vi "Patrick Builder.vi"() -> ()   [LabVIEW 2019, in "Build.lvlib"]
uses:
  Build.lvlib
  <vilib>/Utility/sysdir.llb/System Directory Type.ctl
  Typedefs/Build Type--enum.ctl
  <vilib>/Hampel Software Engineering/Git API/Git API/GIT-api.lvclass
  <vilib>/Utility/file.llb/Read Delimited Spreadsheet (string).vi
  <vilib>/Utility/file.llb/Write Delimited Spreadsheet (string).vi
  <vilib>/regexp/Match Regular Expression.xnode
  <vilib>/JKI/VIPM API/VIPM API_vipm_api.lvlib
  VIPM/VIPM.lvlib
  Git/Git.lvclass
  <userlib>/_OpenG.lib/array/array.llb/Index 1D Array Elements (Path)__ogtk.vi
panel:
  in  "Open Repo":bool
  out "Mode":string
  in  "Edit build.cfg":bool
  in  "Edit Inno.iss":bool
  in  "Init Inno":bool
  in  "BAT File":path
  in  "Execute .bat":bool
  out "Output":string
  in  "Minor +1":bool
  in  "BAT":bool
  out "tag prefix":string caption="tag prefix (level1/level2)"
  in  "Edit File List":bool
  in  "Clear Notes":bool
  in  "Release Notes":string
  in  "Append Notes":bool
  in  "Patch +1":bool
  out "Selected File List":string
  out "Publish":bool
  in  "Open List":bool
  out "Build":bool
  in  "Preview":bool
  out "Status":string
  in  "File List":i32[](listbox)
  out "Package Builder":string
  # "Repository Config"
  # "Global Options (Applied to all Files)"
  # "Release Version"
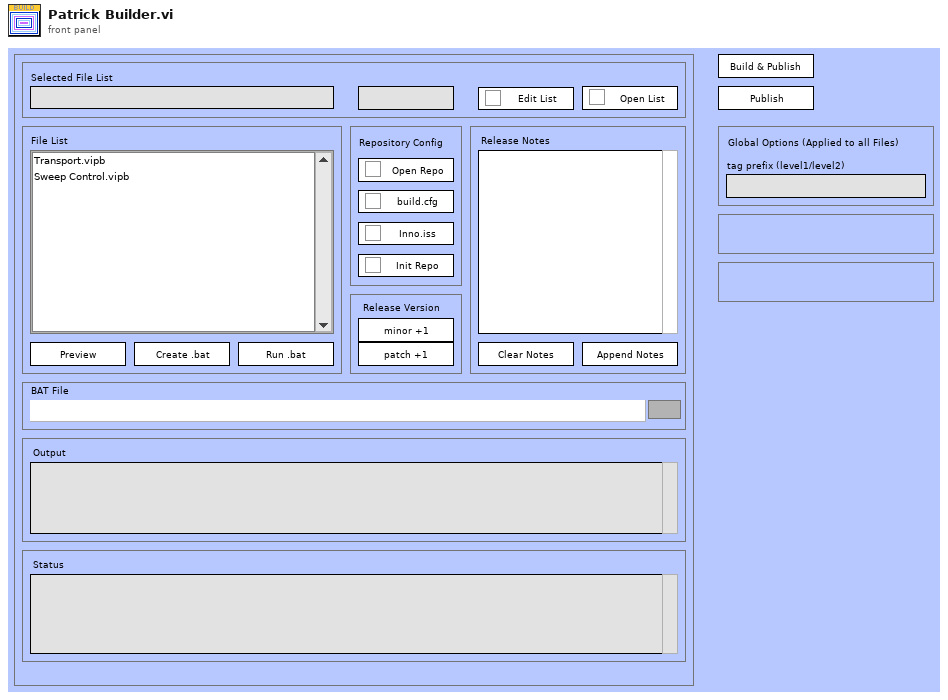
[diagram p1: front panel]
types:
  T1 = enum32{"Invalid", "Standard", "Closed", "Hidden", "Minimized", "Maximized"}
  T2 = enum32{"invalid app kind", "Development System", "Run Time System", "Student Edition", "Embedded LabVIEW", "Evaluation", "Custom"}
  T3 = enum8{"Enabled", "Disabled", "Disabled and Grayed Out"}
  T4 = typedef "Build.lvlib/Build Type--enum.ctl" = enum16{"Project (lvproj)", "Build Spec (vipb)", "Package (vip)"}
  T5 = cluster{"Core":cluster{"Current VI Reference":refnum<vi>, "Close Panel on Exit?":bool}, "lvproj paths":path[], "vipb paths":path[], "vip paths":path[], "selected paths":path[], "repository paths":path[], "path to open":path, ".bat path":path, "config folder":path, "config path":path, "Mode":T4, "git-api":refnum<class "GIT-api.lvclass">}
  T6 = typedef "System Directory Type.ctl" = i32
  T7 = cluster{"Current VI Reference":refnum<vi>, "Close Panel on Exit?":bool}
  T8 = typedef "VIPM API_vipm_api.lvlib/VI Package Build Spec Data Cluster_vipm_api.ctl" = cluster{"Package Version":T9, "Product Name":string, "Company Name":string, "Author Name (Person or Company)":string, "Product Homepage (URL)":string, "Legal Copyright":string, "License Agreement Name":string, "Product Description Summary":string, "Product Description":string, "Release Notes - Change Log":string}
  T9 = typedef "VIPM API_vipm_api.lvlib/Version Info Cluster_vipm_api.ctl" = cluster{"major":u32, "minor":u32, "patch":u32, "build":u32}
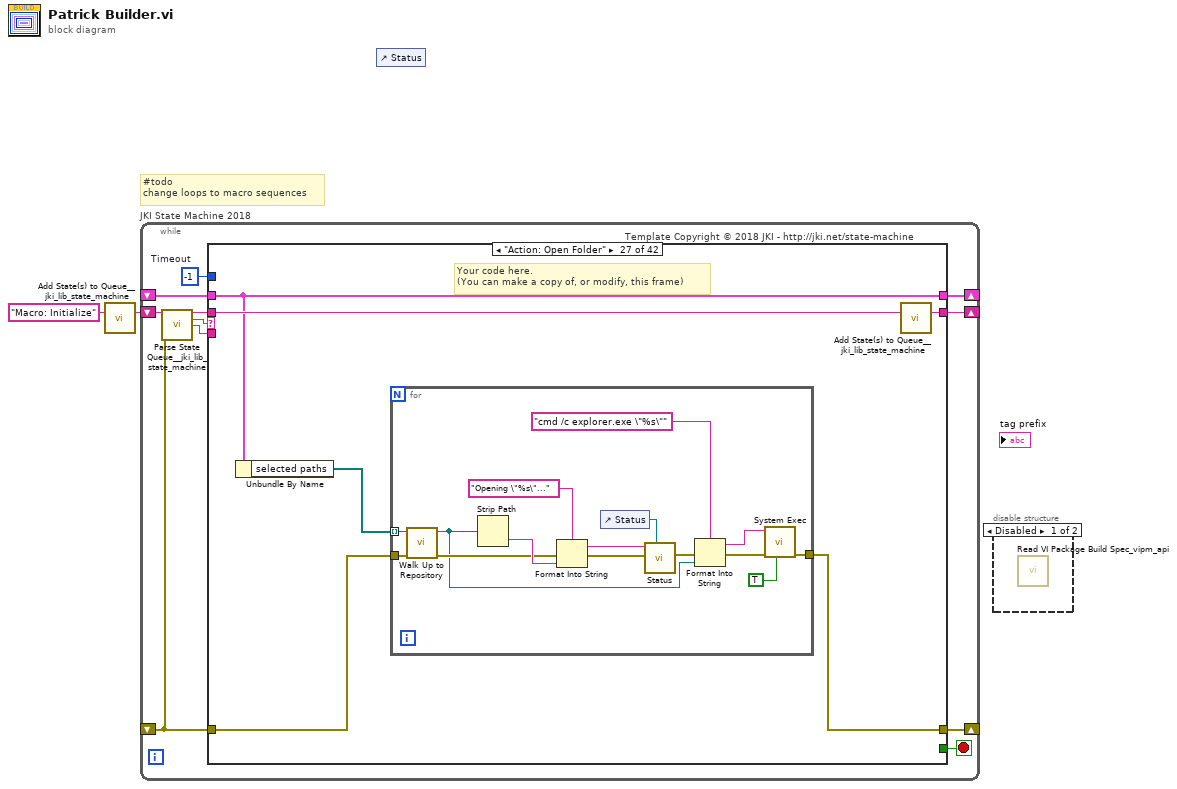
[diagram p0: block diagram]
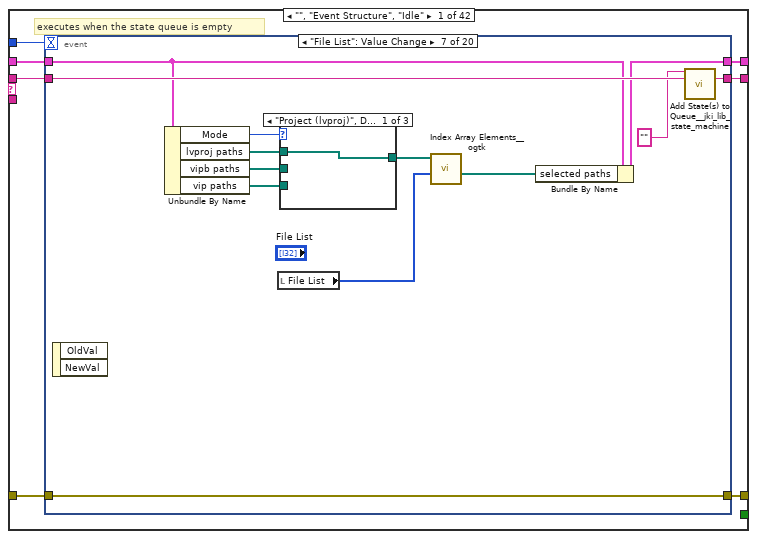
[diagram p3: hidden frame]
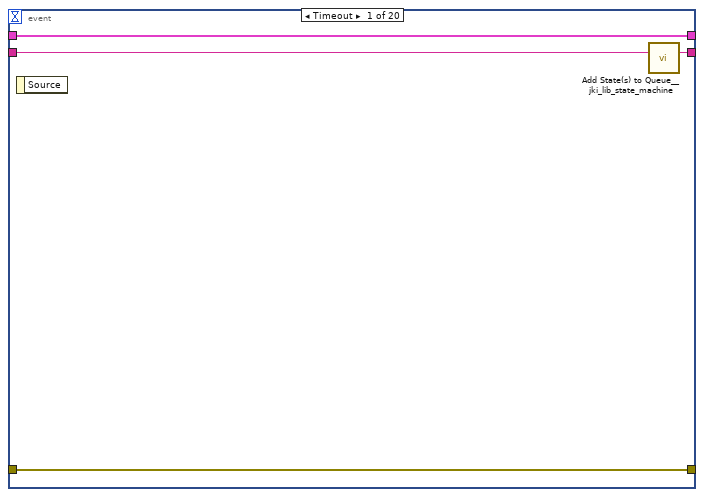
[diagram p4: hidden frame]
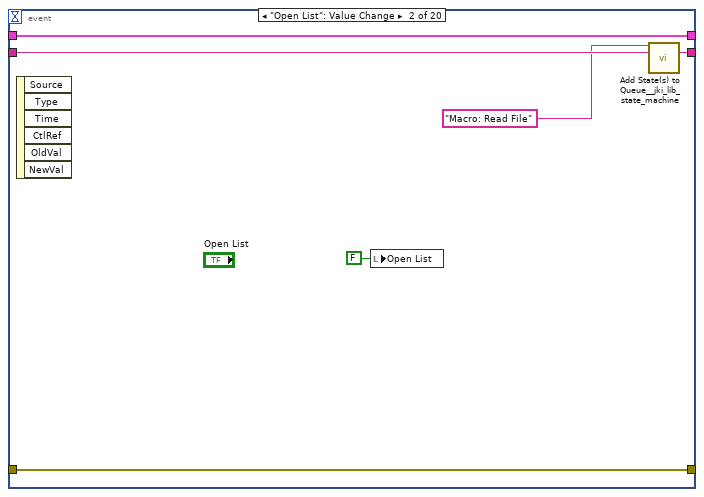
[diagram p5: hidden frame]
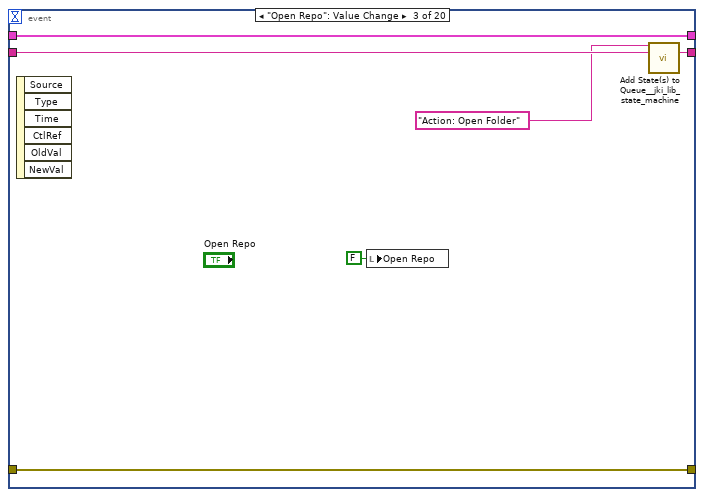
[diagram p6: hidden frame]
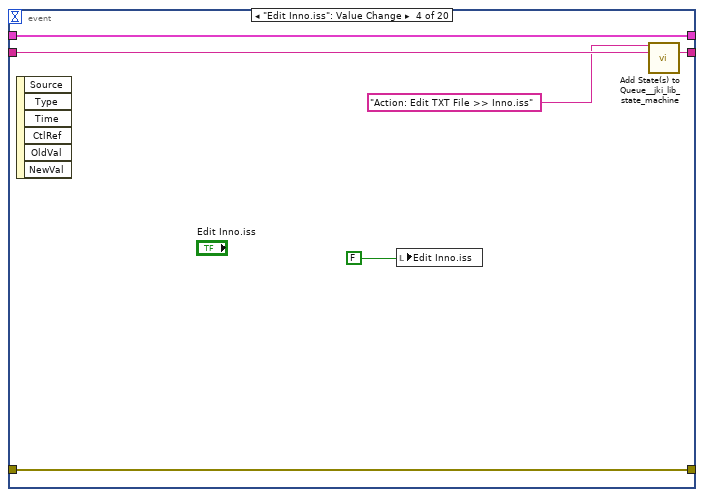
[diagram p7: hidden frame]
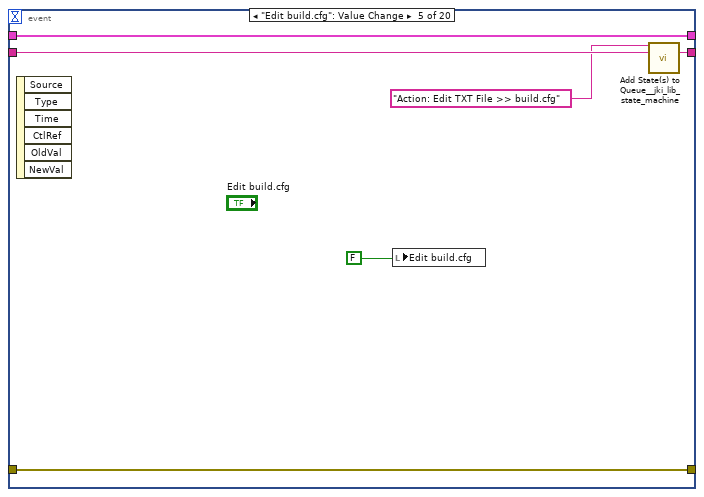
[diagram p8: hidden frame]
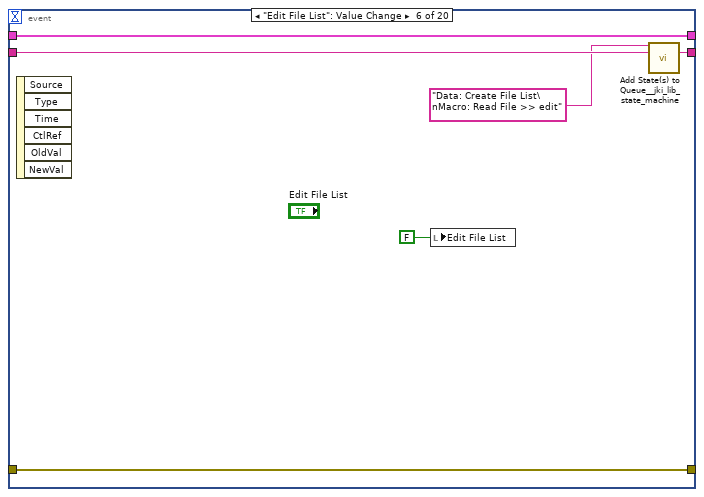
[diagram p9: hidden frame]
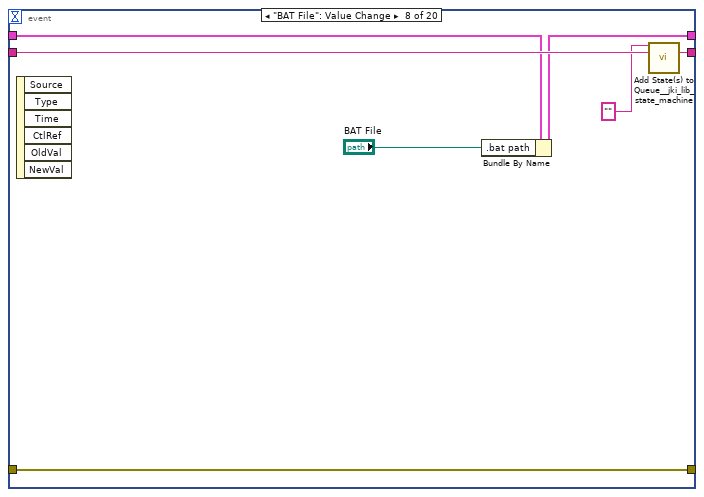
[diagram p12: hidden frame]
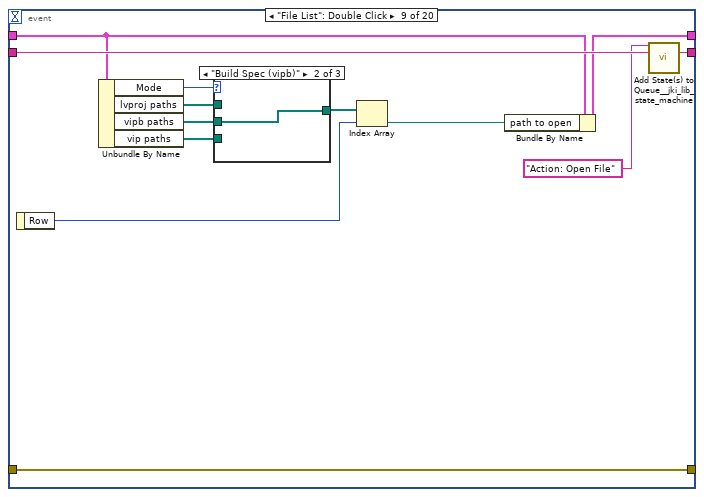
[diagram p13: hidden frame]
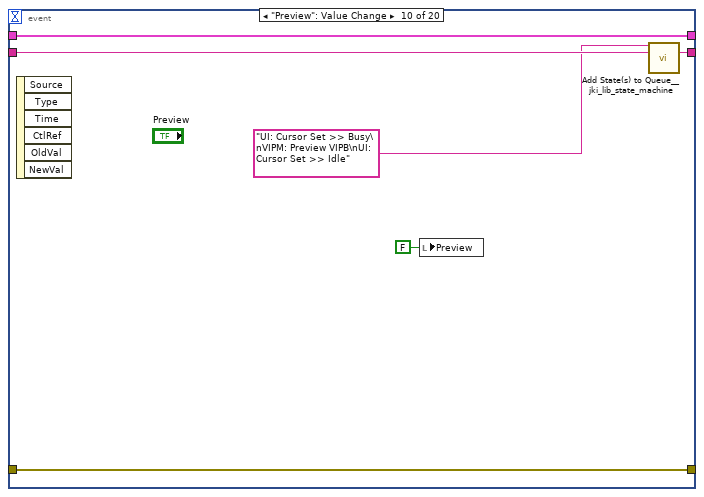
[diagram p16: hidden frame]
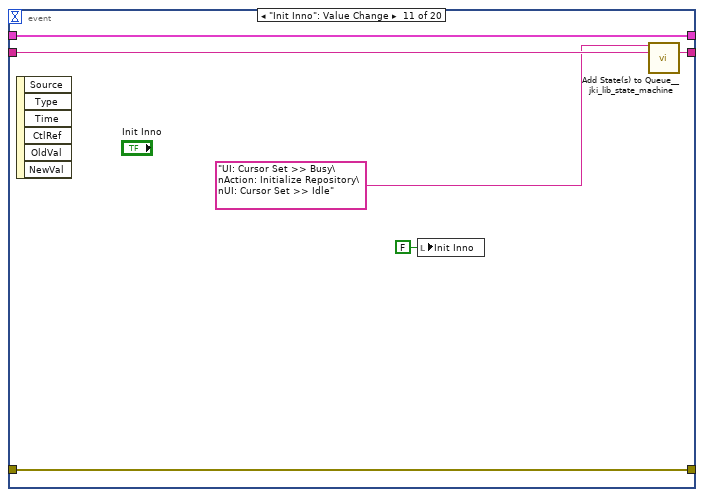
[diagram p17: hidden frame]
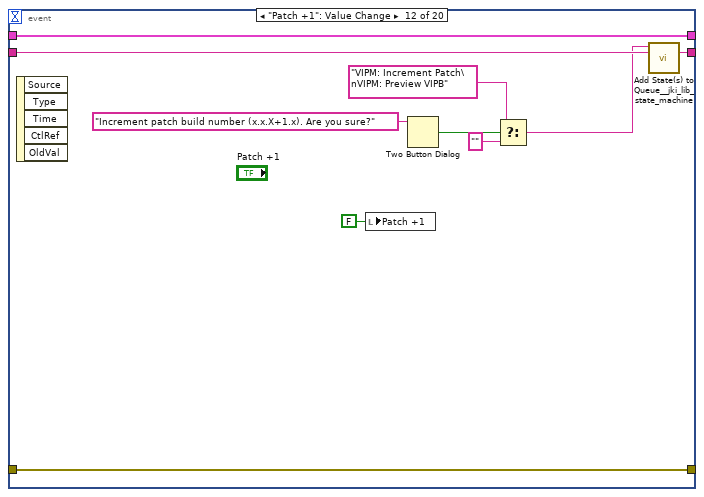
[diagram p18: hidden frame]
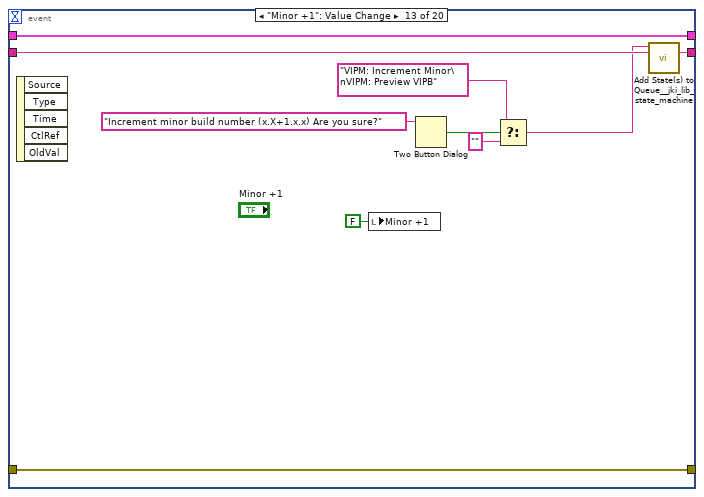
[diagram p19: hidden frame]
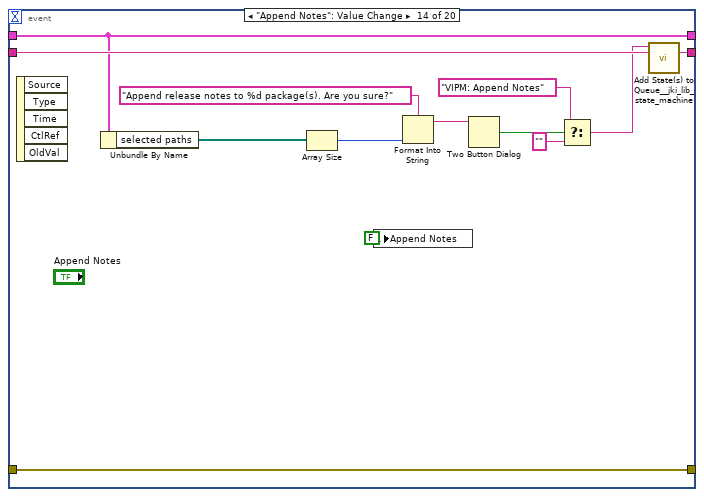
[diagram p20: hidden frame]
diagram:
  # "#todo\nchange loops to macro sequences"
  n1 = call <vilib>:"Add State(s) to Queue__jki_lib_state_machine.vi"("State(s) in (\"\")"="Macro: Initialize") -> ("States Out"=w2:string)  [unwired: 14 in]
  n2 = while "JKI State Machine 2018" {
    shift-right: [w7] -> _
    shift-left: _ -> [w6]
    shift-right: [w10] -> _
    shift-left: _ -> [w4]
    shift-right: [w9] -> _
    shift-left: w2 -> [w11]
    stop <- w8 stop-if-true
    w5 = -1  # Timeout
    # "Template Copyright © 2018 JKI - http://jki.net/state-machine"
    n3 = call <vilib>:"Parse State Queue__jki_lib_state_machine.vi"("State Queue"=w11, "Error In (no error)"=w4) -> ("Remaining States"=w13:string, "Current State"=w3:string, "Arguments"=w12:string)  [unwired: 11 in]
    n4 = case shown="\"Action: Open Folder\"" w3 {
      selector: w3 -> [_ _ w193 _ _ _ _ _ _ _ _ _ _ _ _ _ _ _ _ _ _ _ _ _ _ _ _ _ _ _ _ _ _ _ _ _ _ _ _ _ _ _]
      tunnel: w13 -> [w20 w192 w197 w216 w223 w232 w236 w260 w266 w276 w298 w316 w348 w382 w386 w400 w415 w437 w450 w461 w530 w535 w545 w555 w559 w575 w581 w609 w627 w646 w655 w672 w686 w703 w724 w746 w778 w800 w822 w954 w976 w980]
      tunnel: w12 -> [_ _ _ _ _ _ _ _ _ _ _ _ _ _ _ _ _ _ w445 w455 _ _ w536 _ _ _ _ _ w622 _ _ _ _ _ _ _ _ _ _ _ _ _]
      tunnel: w6 -> [w18 w189 w195 w209 w220 w230 w233 _ w261 w270 w294 w310 w337 w380 w383 w390 w412 w432 w448 w457 w527 w532 w542 w552 w556 w573 w579 w607 w625 w643 w653 w670 w684 w701 w722 w743 w769 w790 w812 w952 w973 w977]
      tunnel: [w17 w190 w199 w213 errorcluster {"status"=FALSE, "code"=0, "source"=""} ("error out") w229 w234 w253 w262 w274 w293 w313 w338 w376 w384 w398 w413 w435 w446 w458 w528 w533 w543 w553 w557 w572 w577 w603 w623 w644 w648 w668 w682 w695 w715 w737 w772 w788 w801 w950 w974 w978] -> w10
      tunnel: w4 -> [w16 w190 w198 w213 w218 w229 w234 w252 w263 w274 w291 w314 w345 w377 w384 w397 w413 w435 w447 w459 w528 w533 w543 w553 w557 w571 w578 w606 w624 w644 w652 w669 w683 w700 w721 w738 w773 w795 w820 w948 w974 w978]
      tunnel: [w19 w191 w196 w215 w222 w231 w235 w259 w265 w275 w297 w315 w347 w381 w385 w399 w414 w436 w449 w460 w529 w534 w544 w554 w558 w574 w580 w608 w626 w645 w654 w671 w685 w702 w723 w745 w777 w799 w821 w953 w975 w979] -> w9
      tunnel: [_ _ _ _ _ TRUE _ _ _ _ _ _ _ _ _ _ _ _ _ _ _ _ _ _ _ _ _ _ _ _ _ _ _ _ _ _ _ _ _ _ _ _] -> w8
      tunnel: [w15 w189 w195 w214 w220 w230 w233 w258 w261 w272 w295 w312 w336 w380 w383 w390 w412 w432 w448 w457 w527 w532 w542 w552 w556 w573 w579 w607 w625 w643 w653 w670 w684 w701 w722 w744 w770 w791 w813 w952 w973 w977] -> w7
      tunnel: w5 -> [w14 _ _ _ _ _ _ _ _ _ _ _ _ _ _ _ _ _ _ _ _ _ _ _ _ _ _ _ _ _ _ _ _ _ _ _ _ _ _ _ _ _]
      frame "", "Event Structure", "Idle" {
        # "executes when the state queue is empty"
        n5 = event shown="[6] \"File List\": Value Change" {
          selector: _ -> [_ _ _ _ _ _ _ _ _ _ _ _ _ _ _ _ _ _ _ _]
          dyn-events: _ -> [_ _ _ _ _ _ _ _ _ _ _ _ _ _ _ _ _ _ _ _]
          timeout: w14 -> [_ _ _ _ _ _ _ _ _ _ _ _ _ _ _ _ _ _ _ _]
          tunnel: w20 -> [w24 w30 w36 w42 w48 w54 w67 w77 w90 w99 w105 w115 w125 w138 w151 w164 w170 w176 w182 w188]
          tunnel: [w23 w29 w35 w41 w47 w53 w66 w76 w89 w98 w104 w114 w124 w137 w150 w163 w169 w175 w181 w187] -> w19
          tunnel: w18 -> [w21 w26 w32 w38 w44 w50 w64 w74 w79 w96 w102 w112 w122 w130 w143 w157 w167 w173 w179 w185]
          tunnel: [w22 w27 w33 w39 w45 w51 w65 w75 w88 w97 w103 w113 w123 w136 w149 w162 w168 w174 w180 w186] -> w17
          tunnel: w16 -> [w22 w27 w33 w39 w45 w51 w65 w75 w88 w97 w103 w113 w123 w136 w149 w162 w168 w174 w180 w186]
          tunnel: [w21 w26 w32 w38 w44 w50 w63 w73 w87 w96 w102 w112 w122 w130 w143 w157 w167 w173 w179 w185] -> w15
          event Timeout {
            n6 = event-data() -> ()  [unwired: 1 in, 1 out]
            n7 = call <vilib>:"Add State(s) to Queue__jki_lib_state_machine.vi"("State(s) in (\"\")"=w24) -> ("States Out"=w23:string)  [unwired: 14 in]
          }
          event "Open List": Value Change {
            n8 = event-data() -> ()  [unwired: 1 in, 6 out]
            n9 = local write "Open List"(FALSE ("Open List")) -> ()
            n10 = call <vilib>:"Add State(s) to Queue__jki_lib_state_machine.vi"("State(s) in Front (\"\")"="Macro: Read File" ("State(s) in Front (\"\")"), "State(s) in (\"\")"=w30) -> ("States Out"=w29:string)  [unwired: 13 in]
          }
          event "Open Repo": Value Change {
            n11 = event-data() -> ()  [unwired: 1 in, 6 out]
            n12 = local write "Open Repo"(FALSE ("Open List")) -> ()
            n13 = call <vilib>:"Add State(s) to Queue__jki_lib_state_machine.vi"("State(s) in Front (\"\")"="Action: Open Folder" ("State(s) in Front (\"\")"), "State(s) in (\"\")"=w36) -> ("States Out"=w35:string)  [unwired: 13 in]
          }
          event "Edit Inno.iss": Value Change {
            n14 = event-data() -> ()  [unwired: 1 in, 6 out]
            n15 = local write "Edit Inno.iss"(FALSE ("Open List")) -> ()
            n16 = call <vilib>:"Add State(s) to Queue__jki_lib_state_machine.vi"("State(s) in Front (\"\")"="Action: Edit TXT File >> Inno.iss" ("State(s) in Front (\"\")"), "State(s) in (\"\")"=w42) -> ("States Out"=w41:string)  [unwired: 13 in]
          }
          event "Edit build.cfg": Value Change {
            n17 = event-data() -> ()  [unwired: 1 in, 6 out]
            n18 = local write "Edit build.cfg"(FALSE ("Open List")) -> ()
            n19 = call <vilib>:"Add State(s) to Queue__jki_lib_state_machine.vi"("State(s) in Front (\"\")"="Action: Edit TXT File >> build.cfg" ("State(s) in Front (\"\")"), "State(s) in (\"\")"=w48) -> ("States Out"=w47:string)  [unwired: 13 in]
          }
          event "Edit File List": Value Change {
            n20 = event-data() -> ()  [unwired: 1 in, 6 out]
            n21 = local write "Edit File List"(FALSE ("Create File List")) -> ()
            n22 = call <vilib>:"Add State(s) to Queue__jki_lib_state_machine.vi"("State(s) in Front (\"\")"="Data: Create File List\nMacro: Read File >> edit" ("State(s) in Front (\"\")"), "State(s) in (\"\")"=w54) -> ("States Out"=w53:string)  [unwired: 13 in]
          }
          event "File List": Value Change {
            n23 = event-data() -> ()  [unwired: 1 in, 2 out]
            n24 = Unbundle By Name(w64) -> ("Mode"=w60:T4, "lvproj paths"=w58:path[], "vipb paths"=w57:path[], "vip paths"=w59:path[])
            n25 = local read "File List"() -> (w56:i32[])
            n26 = case shown="\"Project (lvproj)\", Default" w60 {
              tunnel: [w68 w69 w70] -> w55
              tunnel: w59 -> [_ _ w70]
              tunnel: w58 -> [w68 _ _]
              tunnel: w57 -> [_ w69 _]
              frame "Project (lvproj)", Default {
              }
              frame "Build Spec (vipb)" {
              }
              frame "Package (vip)" {
              }
            }
            n27 = call-poly <userlib>:"Index Array Elements__ogtk.vi"("indices"=w56, "array"=w55) -> ("elements"=w62:path[])  [unwired: 9 in]
            n28 = Bundle By Name(cluster=w64, "selected paths"=w62) -> (w63:T5)
            n29 = call <vilib>:"Add State(s) to Queue__jki_lib_state_machine.vi"("State(s) in Front (\"\")"="" ("State(s) in Front (\"\")"), "State(s) in (\"\")"=w67) -> ("States Out"=w66:string)  [unwired: 13 in]
          }
          event "BAT File": Value Change {
            n30 = event-data() -> ()  [unwired: 1 in, 6 out]
            n31 = Bundle By Name(cluster=w74, ".bat path"="BAT File") -> (w73:T5)
            n32 = call <vilib>:"Add State(s) to Queue__jki_lib_state_machine.vi"("State(s) in Front (\"\")"="" ("State(s) in Front (\"\")"), "State(s) in (\"\")"=w77) -> ("States Out"=w76:string)  [unwired: 13 in]
          }
          event "File List": Double Click {
            n33 = event-data() -> ("Row"=w84:i32)  [unwired: 1 in]
            n34 = Unbundle By Name(w79) -> ("Mode"=w83:T4, "lvproj paths"=w81:path[], "vipb paths"=w80:path[], "vip paths"=w82:path[])
            n35 = case shown="\"Build Spec (vipb)\"" w83 {
              tunnel: [w91 w92 w93] -> w78
              tunnel: w82 -> [_ _ w93]
              tunnel: w81 -> [w91 _ _]
              tunnel: w80 -> [_ w92 _]
              frame "Project (lvproj)", Default {
              }
              frame "Build Spec (vipb)" {
              }
              frame "Package (vip)" {
              }
            }
            n36 = Index Array(array=w78, index=w84) -> (element=w86:path)
            n37 = Bundle By Name(cluster=w79, "path to open"=w86) -> (w87:T5)
            n38 = call <vilib>:"Add State(s) to Queue__jki_lib_state_machine.vi"("State(s) in Front (\"\")"="Action: Open File" ("State(s) in Front (\"\")"), "State(s) in (\"\")"=w90) -> ("States Out"=w89:string)  [unwired: 13 in]
          }
          event "Preview": Value Change {
            n39 = event-data() -> ()  [unwired: 1 in, 6 out]
            n40 = local write "Preview"(FALSE ("Preview")) -> ()
            n41 = call <vilib>:"Add State(s) to Queue__jki_lib_state_machine.vi"("State(s) in Front (\"\")"="UI: Cursor Set >> Busy\nVIPM: Preview VIPB\nUI: Cursor Set >> Idle" ("State(s) in Front (\"\")"), "State(s) in (\"\")"=w99) -> ("States Out"=w98:string)  [unwired: 13 in]
          }
          event "Init Inno": Value Change {
            n42 = event-data() -> ()  [unwired: 1 in, 6 out]
            n43 = local write "Init Inno"(FALSE ("Preview")) -> ()
            n44 = call <vilib>:"Add State(s) to Queue__jki_lib_state_machine.vi"("State(s) in Front (\"\")"="UI: Cursor Set >> Busy\nAction: Initialize Repository\nUI: Cursor Set >> Idle" ("State(s) in Front (\"\")"), "State(s) in (\"\")"=w105) -> ("States Out"=w104:string)  [unwired: 13 in]
          }
          event "Patch +1": Value Change {
            n45 = event-data() -> ()  [unwired: 1 in, 5 out]
            n46 = local write "Patch +1"(FALSE ("Patch +1")) -> ()
            n47 = Two Button Dialog(message="Increment patch build number (x.x.X+1.x). Are you sure?") -> (T button?=w110:bool)  [unwired: 2 in]
            n48 = Select(t="VIPM: Increment Patch\nVIPM: Preview VIPB" ("State(s) in Front (\"\")"), s=w110, f="") -> (s? t:f=w108:string)
            n49 = call <vilib>:"Add State(s) to Queue__jki_lib_state_machine.vi"("State(s) in Front (\"\")"=w108, "State(s) in (\"\")"=w115) -> ("States Out"=w114:string)  [unwired: 13 in]
          }
          event "Minor +1": Value Change {
            n50 = event-data() -> ()  [unwired: 1 in, 5 out]
            n51 = local write "Minor +1"(FALSE ("Patch +1")) -> ()
            n52 = Two Button Dialog(message="Increment minor build number (x.X+1.x.x) Are you sure?") -> (T button?=w120:bool)  [unwired: 2 in]
            n53 = Select(t="VIPM: Increment Minor\nVIPM: Preview VIPB" ("State(s) in Front (\"\")"), s=w120, f="") -> (s? t:f=w118:string)
            n54 = call <vilib>:"Add State(s) to Queue__jki_lib_state_machine.vi"("State(s) in Front (\"\")"=w118, "State(s) in (\"\")"=w125) -> ("States Out"=w124:string)  [unwired: 13 in]
          }
          event "Append Notes": Value Change {
            n55 = event-data() -> ()  [unwired: 1 in, 5 out]
            n56 = Unbundle By Name(w130) -> ("selected paths"=w128:path[])
            n57 = Array Size(array=w128) -> (size(s)=w129:i32)
            n58 = local write "Append Notes"(FALSE ("Patch +1")) -> ()
            n59 = Format Into String(format string="Append release notes to %d package(s). Are you sure?" ("message"), w129) -> (resulting string=w132:string)  [unwired: 2 in, 1 out]
            n60 = Two Button Dialog(message=w132) -> (T button?=w135:bool)  [unwired: 2 in]
            n61 = Select(t="VIPM: Append Notes" ("State(s) in Front (\"\")"), s=w135, f="") -> (s? t:f=w133:string)
            n62 = call <vilib>:"Add State(s) to Queue__jki_lib_state_machine.vi"("State(s) in Front (\"\")"=w133, "State(s) in (\"\")"=w138) -> ("States Out"=w137:string)  [unwired: 13 in]
          }
          event "Clear Notes": Value Change {
            n63 = event-data() -> ()  [unwired: 1 in, 6 out]
            n64 = Unbundle By Name(w143) -> ("selected paths"=w141:path[])
            n65 = local write "Clear Notes"(FALSE ("Patch +1")) -> ()
            n66 = Array Size(array=w141) -> (size(s)=w142:i32)
            n67 = Format Into String(format string="Clear release notes from %d package(s). Are you sure?" ("message"), w142) -> (resulting string=w145:string)  [unwired: 2 in, 1 out]
            n68 = Two Button Dialog(message=w145) -> (T button?=w148:bool)  [unwired: 2 in]
            n69 = Select(t="VIPM: Clear Notes" ("State(s) in Front (\"\")"), s=w148, f="") -> (s? t:f=w146:string)
            n70 = call <vilib>:"Add State(s) to Queue__jki_lib_state_machine.vi"("State(s) in Front (\"\")"=w146, "State(s) in (\"\")"=w151) -> ("States Out"=w150:string)  [unwired: 13 in]
          }
          event "Build": Value Change {
            n71 = event-data() -> ()  [unwired: 1 in, 6 out]
            n72 = Unbundle By Name(w157) -> ("selected paths"=w153:path[])
            n73 = local write "Build"(FALSE ("Patch +1")) -> ()
            n74 = Array Size(array=w153) -> (size(s)=w154:i32)
            n75 = Format Into String(format string="You have chosen to build and publish %d package(s). Are you sure?" ("message"), w154) -> (resulting string=w156:string)  [unwired: 2 in, 1 out]
            n76 = Two Button Dialog(message=w156) -> (T button?=w161:bool)  [unwired: 2 in]
            n77 = Select(t="VIPM: Build\nUI: Disable Buttons\nUI: Enable Buttons\nVIPM: Publish" ("State(s) in Front (\"\")"), s=w161, f="") -> (s? t:f=w158:string)
            n78 = call <vilib>:"Add State(s) to Queue__jki_lib_state_machine.vi"("State(s) in Front (\"\")"=w158, "State(s) in (\"\")"=w164) -> ("States Out"=w163:string)  [unwired: 13 in]
          }
          event "Publish": Value Change {
            n79 = event-data() -> ()  [unwired: 1 in, 6 out]
            n80 = local write "Publish"(FALSE ("Patch +1")) -> ()
            n81 = call <vilib>:"Add State(s) to Queue__jki_lib_state_machine.vi"("State(s) in Front (\"\")"="VIPM: Publish" ("State(s) in Front (\"\")"), "State(s) in (\"\")"=w170) -> ("States Out"=w169:string)  [unwired: 13 in]
          }
          event "BAT": Value Change {
            n82 = event-data() -> ()  [unwired: 1 in, 6 out]
            n83 = local write "BAT"(FALSE ("Patch +1")) -> ()
            n84 = call <vilib>:"Add State(s) to Queue__jki_lib_state_machine.vi"("State(s) in Front (\"\")"="VIPM: Create Build File\nVIPM: Create Build All File" ("State(s) in Front (\"\")"), "State(s) in (\"\")"=w176) -> ("States Out"=w175:string)  [unwired: 13 in]
          }
          event "Execute .bat": Value Change {
            n85 = event-data() -> ()  [unwired: 1 in, 6 out]
            n86 = local write "Execute .bat"(FALSE ("Patch +1")) -> ()
            n87 = call <vilib>:"Add State(s) to Queue__jki_lib_state_machine.vi"("State(s) in Front (\"\")"="VIPM: Run BAT File\nVIPM: Publish" ("State(s) in Front (\"\")"), "State(s) in (\"\")"=w182) -> ("States Out"=w181:string)  [unwired: 13 in]
          }
          event Panel Close? {
            # "Discard the event because we'll close the front panel ourselves in Macro: Exit"
            # "Close Panel button (pressed) Event\n(this executes Macro: Exit to terminate the VI)"
            n88 = event-data() -> ()  [unwired: 1 in, 1 out]
            n89 = event-data("Discard?"=TRUE) -> ()  [unwired: 1 in, 1 out]
            n90 = call <vilib>:"Add State(s) to Queue__jki_lib_state_machine.vi"("State(s) in Front (\"\")"="Macro: Exit", "State(s) in (\"\")"=w188) -> ("States Out"=w187:string)  [unwired: 13 in]
          }
        }
      }
      frame "---------- Core ----------" {
        # "Do not put any code in this frame.\n(it is a separator no-op)"
        n91 = call <vilib>:"Add State(s) to Queue__jki_lib_state_machine.vi"("State(s) in (\"\")"=w192) -> ("States Out"=w191:string)  [unwired: 14 in]
      }
      frame Default {
        w202 = 42 items=["No error", "Argument error", "Memory is full", "Out of zone", "End of file", "File already open", "Generic file I/O error", "File not found", "File permission error", "Disk is full", "Duplicate path", "Too many files open", "System feature not enabled", "Resource file not found", "Cannot add resource", "Resource not found", "Image not found", "Image memory error", "Pen does not exist", "Config type invalid", "Config token not found", "Config parse error", "Config memory error", "Bad external code format", "Bad external code offset", "External code not present", "Null window", "Destroy window error", "Null menu", "Print aborted", "Bad print record", "Print driver error", "Windows error during printing", "Memory error during printing", "Print dialog error", "Generic print error", "Invalid device refnum", "Device not found", "Device parameter error", "Device unit error", "Cannot open device", "Device call aborted", "Generic error", "Cancelled by user", "Object ID too low", "Object ID too high", "Object not in heap", "Unknown heap", "Unknown object (invalid DefProc)", "Unknown object (DefProc not in table)", "Message out of range", "Invalid (null) method", "Unknown message", "Manager call not supported", "Bad address", "Network operation in progress", "Network operation timed out", "Connection is busy", "Network attribute not supported", "Network error", "Address in use", "System out of memory", "Connection aborted", "Connection refused", "Not connected", "Already connected", "Connection closed", "Initialization error (interapplication manager)", "Bad occurrence", "Wait on unbound occurrence handler", "Occurrence queue overflow", "Datalog type conflict", "Unused", "Unrecognized type (interapplication manager)", "Memory corrupt", "Failed to make temporary DLL", "Old CIN version", "Drag socket not found", "Failed to load drop-object", "Failed to register OLE object", "Failed to release OLE object", "Format specifier type mismatch", "Unknown format specifier", "Too few format specifiers", "Too many format specifiers", "Scan failed", "Newer CIN version", "Error converting to variant", "Runtime menu error", "Password tampered", "Variant attribute not found", "Incompatible variant data type", "Event data is not available", "Event Store is not present", "Occurrence is not found", "Event Queue is not created", "Event info is not available", "Refnum passed is NULL", "Error retrieving Class GUID", "Error retrieving CoClass GUID", "Error retrieving TypeLib GUID.", "Bad built application magic bytes.", "Specific driver is different from the specific driver associated with the Logical Name.", "There is no session opened to the class driver.", "Max Error", "MAX - Error with config objects", "MAX - Error loading configuration", "MAX - Group not supported"]
        # "Current State"
        # "Do not delete, rename, or modify this frame.\n(this is used to capture unhandled states and typos)"
        # "Handle mistyped state name (developer tool)"
        n92 = Format Into String(format string="Software Exception: Unhandled State \"%s\"." ("message"), error in=w198, w193) -> (resulting string=w201:string, error out=w200:errorcluster)  [unwired: 1 in]
        n93 = call <vilib>:"Error Cluster From Error Code.vi"("show call chain? (False)"=TRUE, "error in (no error)"=w200, "error message (\"\")"=w201, "error code (0)"=w202) -> ("error out"=w199:errorcluster)  [unwired: 5 in]
        n94 = call <vilib>:"Add State(s) to Queue__jki_lib_state_machine.vi"("State(s) in (\"\")"=w197) -> ("States Out"=w196:string)  [unwired: 14 in]
      }
      frame "Initialize Core Data" {
        # "Do not delete, rename, or modify this frame.\n(this is used to determine panel behavior on exit)"
        # "originally closed?"
        # "exe?"
        # "If panel starts closed or is an EXE, then close it when we exit"
        n95 = property class="VI"() -> ("FP.State"=w206:T1)  [unwired: 2 in, 2 out]
        n96 = property class="App"() -> ("App.Kind"=w212:T2)  [unwired: 2 in, 2 out]
        n97 = control-ref of="Current VI Reference"() -> (w207:refnum<vi>)
        n98 = Equal?(x=w206, y=T1."Closed" ("Front Panel Window:State")) -> (x = y?=w204:bool)
        n99 = Equal?(x=w212, y=T2."Run Time System" ("Application:Kind")) -> (x = y?=w210:bool)
        n100 = Or(x=w204, y=w210) -> (x .or. y?=w208:bool)
        n101 = Bundle By Name(cluster=w209, "Core.Current VI Reference"=w207, "Core.Close Panel on Exit?"=w208) -> (w214:T5)
        n102 = call <vilib>:"Add State(s) to Queue__jki_lib_state_machine.vi"("State(s) in (\"\")"=w216) -> ("States Out"=w215:string)  [unwired: 14 in]
      }
      frame "Error Handler" {
        # "Unhandled Error -- Display it"
        # "Handle any errors here.\nYou can also output any states to clean-up after errors occur"
        # "Clear error"
        n103 = case shown="Default" w218 {
          selector: w218 -> [w224 w225 _]
          tunnel: [w224 w225 w226] -> w217
          frame No Error {
          }
          frame Default {
          }
          frame Error {
            n104 = property on="Open List" class="Bool (strict)"("Val(Sgnl)"=TRUE) -> (error out=w226:errorcluster)  [unwired: 2 in, 1 out]
          }
        }
        n105 = call <vilib>:"General Error Handler.vi"("error in (no error)"=w217) -> ()  [unwired: 10 in, 5 out]
        n106 = call <vilib>:"Add State(s) to Queue__jki_lib_state_machine.vi"("State(s) in Front (\"\")"="/* Post Error States", "State(s) in (\"\")"=w223) -> ("States Out"=w222:string)  [unwired: 13 in]
      }
      frame "Exit" {
        # "Do not put any code in this frame.\n(No errors that occur here will be handled.)"
        n107 = call <vilib>:"Add State(s) to Queue__jki_lib_state_machine.vi"("State(s) in (\"\")"=w232) -> ("States Out"=w231:string)  [unwired: 14 in]
      }
      frame "---------- Data ----------" {
        # "Do not put any code in this frame.\n(It is a separator no-op. You can make a copy of this frame to create a new Data frame)"
        n108 = call <vilib>:"Add State(s) to Queue__jki_lib_state_machine.vi"("State(s) in (\"\")"=w236) -> ("States Out"=w235:string)  [unwired: 14 in]
      }
      frame "Data: Initialize" {
        w237 = path ""  # .bat path
        w240 = path ""  # config folder
        w241 = path[] []  # repository paths
        w242 = path ""  # path to open
        w243 = refnum<class "GIT-api.lvclass"> refnum  # git-api
        w244 = Build_Type--enum."Project (lvproj)"  # Mode
        w248 = T6 3 items=["User Home"=0, "User Desktop"=1, "User Documents"=2, "User Application Data"=3, "User Preferences"=4, "User Temporary"=5, "Public Documents"=6, "Public Application Data"=7, "Public Preferences"=8, "Public Cache"=13, "System Core Libraries"=9, "System Installed Libraries"=10, "Application Files"=11, "Boot Volume Root"=12] ("system directory type")
        w249 = path[] []  # lvproj paths
        w250 = path[] []  # vip paths
        w251 = path[] []  # vipb paths
        w254 = path ""  # config path
        w256 = path[] []  # selected paths
        w257 = T7 {"Current VI Reference"=refnum, "Close Panel on Exit?"=FALSE}  # Core
        # "Initialize the shift-register data, here.\n(data names are defined by what you wire into the bundle function)"
        n109 = call <vilib>:"Get System Directory.vi"("system directory type"=w248) -> ("system directory"=w247:path)  [unwired: 10 in]
        n110 = Build Path(base path=w247, name or relative path="LevyLab\\build-support") -> (appended path=w246:path)
        n111 = call <vilib>:"Create Directory Recursive.vi"("error in (no error)"=w252, "directory"=w246) -> ("error out"=w253:errorcluster, "directory copy"=w239:path)  [unwired: 3 in, 1 out]
        n112 = Variant To Data(type=w240, Variant=w239) -> (data=w238:path)  [unwired: 1 in, 1 out]
        n113 = Variant To Data(type=w254, Variant=w239) -> (data=w255:path)  [unwired: 1 in, 1 out]
        n114 = Bundle("Core"=w257, "lvproj paths"=w249, "vipb paths"=w251, "vip paths"=w250, "selected paths"=w256, "repository paths"=w241, "path to open"=w242, ".bat path"=w237, "config folder"=w238, "config path"=w255, "Mode"=w244, "git-api"=w243) -> (w258:T5)  [unwired: 1 in]
        n115 = call <vilib>:"Add State(s) to Queue__jki_lib_state_machine.vi"("State(s) in (\"\")"=w260) -> ("States Out"=w259:string)  [unwired: 14 in]
      }
      frame "Data: Cleanup" {
        # "Cleanup any data and references, here.\n(this is called automatically, by the Macro: Exit)"
        n116 = Unbundle By Name(w261) -> ("Core.Current VI Reference"=w264:refnum<vi>)
        n117 = Close Reference(reference=w264, error in (no error)=w263) -> (error out=w262:errorcluster)
        n118 = call <vilib>:"Add State(s) to Queue__jki_lib_state_machine.vi"("State(s) in (\"\")"=w266) -> ("States Out"=w265:string)  [unwired: 14 in]
      }
      frame "Data: Update Listbox" {
        # "Do not put any code in this frame.\n(It is a separator no-op. You can make a copy of this frame to create a new Data frame)"
        n119 = Unbundle By Name(w270) -> ("Mode"=w271:T4)
        n120 = case shown="\"Package (vip)\"" w271 {
          tunnel: w270 -> [w278 w280 w282]
          tunnel: [w277 w279 w281] -> w269
          frame "Project (lvproj)", Default {
            n121 = Unbundle By Name(w278) -> ("lvproj paths"=w277:path[])
          }
          frame "Build Spec (vipb)" {
            n122 = Unbundle By Name(w280) -> ("vipb paths"=w279:path[])
          }
          frame "Package (vip)" {
            n123 = Unbundle By Name(w282) -> ("vip paths"=w281:path[])
          }
        }
        n124 = for {
          tunnel: w269 -> [w285] mode=indexing
          tunnel: [w284] -> w273 mode=indexing
          tunnel: [w283] -> _ mode=indexing
          i -> [w283]
          n125 = Strip Path(path=w285) -> (name=w284:string)  [unwired: 1 out]
        }
        n126 = Bundle By Name(cluster=w270, "selected paths"=path[] [] ("f")) -> (w272:T5)
        n127 = property on="File List" class="LstBox (strict)"("Item Names"=w273, "Value"=i32[] [] ("File List")) -> ()  [unwired: 2 in, 2 out]
        n128 = call <vilib>:"Add State(s) to Queue__jki_lib_state_machine.vi"("State(s) in (\"\")"=w276) -> ("States Out"=w275:string)  [unwired: 14 in]
      }
      frame "Data: Choose File List" {
        # "Do not put any code in this frame.\n(It is a separator no-op. You can make a copy of this frame to create a new Data frame)"
        n129 = Unbundle By Name(w294) -> ("config path"=w290:path)
        n130 = call "File Dialog2"("start path"=w290, "prompt"="Choose list file to open", "error in"=w291, "pattern (all files)"="*.txt") -> ("selected path"=w287:path, "cancelled"=w289:bool, "error out"=w288:errorcluster)  [unwired: 8 in, 1 out]
        n131 = case shown="False" w289 {
          tunnel: w287 -> [w299 _]
          tunnel: [w303 _] -> w296
          tunnel: [w302 w304] -> w295
          tunnel: w294 -> [w301 w304]
          tunnel: w288 -> [w300 _]
          tunnel: [w300 _] -> w293
          frame False {
            n132 = Bundle By Name(cluster=w301, "config path"=w299) -> (w302:T5)
            n133 = Strip Path(path=w299) -> (name=w303:string)  [unwired: 1 out]
          }
          frame True {
          }
        }
        "Selected File List" <- w296
        n134 = call <vilib>:"Add State(s) to Queue__jki_lib_state_machine.vi"("State(s) in (\"\")"=w298) -> ("States Out"=w297:string)  [unwired: 14 in]
      }
      frame "Data: Create File List" {
        # "Do not put any code in this frame.\n(It is a separator no-op. You can make a copy of this frame to create a new Data frame)"
        n135 = Unbundle By Name(w310) -> ("config path"=w309:path, "Mode"=w308:T4)
        n136 = call "File List Window.vi"("error in"=w314, "File Type"=w308, "Path"=w309) -> ("error out"=w313:errorcluster, "File Type out"=w307:T4, "files out"=w306:path[], "Path out"=w305:path)  [unwired: 5 in]
        n137 = Empty Array?(array=w306) -> (empty?=w311:bool)
        n138 = case shown="False" w311 {
          tunnel: [w319 w332] -> w312
          tunnel: w310 -> [w322 w332]
          tunnel: w307 -> [w317 _]
          tunnel: w306 -> [w321 _]
          tunnel: w305 -> [w318 _]
          frame False {
            n139 = case shown="\"Build Spec (vipb)\"" w317 {
              tunnel: [w325 w328 w331] -> w320
              tunnel: w322 -> [w324 w327 w330]
              tunnel: w321 -> [w323 w326 w329]
              frame "Project (lvproj)" {
                n140 = Bundle By Name(cluster=w324, "lvproj paths"=w323) -> (w325:T5)
              }
              frame "Build Spec (vipb)" {
                n141 = Bundle By Name(cluster=w327, "vipb paths"=w326) -> (w328:T5)
              }
              frame "Package (vip)" {
                n142 = Bundle By Name(cluster=w330, "vip paths"=w329) -> (w331:T5)
              }
            }
            n143 = Bundle By Name(cluster=w320, "Mode"=w317, "config path"=w318) -> (w319:T5)
          }
          frame True {
          }
        }
        n144 = call <vilib>:"Add State(s) to Queue__jki_lib_state_machine.vi"("State(s) in (\"\")"=w316) -> ("States Out"=w315:string)  [unwired: 14 in]
      }
      frame "Data: Read File List" {
        # "Do not put any code in this frame.\n(It is a separator no-op. You can make a copy of this frame to create a new Data frame)"
        n145 = Unbundle By Name(w337) -> ("config path"=w346:path)
        n146 = call-poly <vilib>:"Read Delimited Spreadsheet.vi"("file path (dialog if empty)"=w346, "error in (no error)"=w345, "transpose? (F)"=TRUE, "delimiter (\\t)"="\\n" ("delimiter (\\t)")) -> ("all rows"=w343:string[][], "error out"=w339:errorcluster)  [unwired: 6 in, 4 out]
        n147 = Index Array(array=w343) -> (element=w342:string[])  [unwired: 2 in]
        n148 = String To Path(string=w342) -> (path=w340:path[])
        n149 = for {
          tunnel: w340 -> [w372] mode=indexing
          tunnel: w339 -> [w371]
          tunnel: [w370] -> w338
          tunnel: [w368] -> w335 mode=indexing
          tunnel: [w367] -> w333
          n150 = call <vilib>:"Get File Extension.vi"("error in (no error)"=w371, "file"=w372) -> ("error out"=w370:errorcluster, "lowercase file extension"=w369:string, "dup file"=w368:path)  [unwired: 5 in, 2 out]
          n151 = call "Extension to Mode.vi"("lowercase file extension"=w369) -> ("Mode"=w367:T4)  [unwired: 10 in]
        }
        n152 = Empty Array?(array=w335) -> (empty?=w334:bool)
        n153 = case shown="False" w334 {
          tunnel: [w353 w366] -> w336
          tunnel: w337 -> [w352 w366]
          tunnel: w333 -> [w350 _]
          tunnel: w335 -> [w351 _]
          frame False {
            n154 = case shown="\"Package (vip)\"" w350 {
              selector: w350 -> [w354 w358 w362]
              tunnel: [w357 w361 w365] -> w353
              tunnel: w352 -> [w356 w360 w364]
              tunnel: w351 -> [w355 w359 w363]
              frame "Project (lvproj)" {
                n155 = Bundle By Name(cluster=w356, "lvproj paths"=w355, "Mode"=w354) -> (w357:T5)
              }
              frame "Build Spec (vipb)" {
                n156 = Bundle By Name(cluster=w360, "vipb paths"=w359, "Mode"=w358) -> (w361:T5)
              }
              frame "Package (vip)" {
                n157 = Bundle By Name(cluster=w364, "vip paths"=w363, "Mode"=w362) -> (w365:T5)
              }
            }
            n158 = Format Into String(w350) -> (resulting string=→"Mode":string)  [unwired: 3 in, 1 out]
          }
          frame True {
          }
        }
        n159 = call <vilib>:"Add State(s) to Queue__jki_lib_state_machine.vi"("State(s) in (\"\")"=w348) -> ("States Out"=w347:string)  [unwired: 14 in]
      }
      frame "Data: Save File List" {
        # "Do not put any code in this frame.\n(It is a separator no-op. You can make a copy of this frame to create a new Data frame)"
        n160 = Unbundle By Name(w380) -> ("config path"=w375:path, "vipb paths"=w379:path[])
        n161 = Path To String(path=w379) -> (string=w378:string[])
        n162 = call-poly <vilib>:"Write Delimited Spreadsheet.vi"("file path (dialog if empty)"=w375, "1D data"=w378, "error in (no error)"=w377, "transpose? (no:F)"=TRUE, "delimiter (\\t)"="\\n" ("delimiter (\\t)")) -> ("error out"=w376:errorcluster)  [unwired: 9 in, 1 out]
        n163 = call <vilib>:"Add State(s) to Queue__jki_lib_state_machine.vi"("State(s) in (\"\")"=w382) -> ("States Out"=w381:string)  [unwired: 14 in]
      }
      frame "---------- UI ----------" {
        # "Do not put any code in this frame.\n(It is a separator no-op. You can make a copy of this frame to create a new UI frame)"
        n164 = call <vilib>:"Add State(s) to Queue__jki_lib_state_machine.vi"("State(s) in (\"\")"=w386) -> ("States Out"=w385:string)  [unwired: 14 in]
      }
      frame "UI: Initialize" {
        w392 = "" ("Status")
        # "Initialize the User Interface, here.\n(this is called automatically, by the Macro: Init)"
        n165 = Unbundle By Name(w390) -> ("config path"=w389:path)
        n166 = Build Path(base path=w389, name or relative path="scripts") -> (appended path=w387:path)
        n167 = call <userlib>:"MGI Get Executable Version.vi"() -> ("Version"=w395:string)  [unwired: 7 in]
        n168 = local write "BAT File"(path "" (".bat File")) -> ()
        n169 = Format Into String(format string="Patrick Builder v%s - build-support 1.11.4", w395) -> (resulting string=→"Package Builder":string)  [unwired: 2 in, 1 out]
        n170 = call <userlib>:"Fit VI window to Largest Dec__ogtk.vi"("error in (no error)"=w397, "border spacing (2 px)"=0) -> ("error out"=w398:errorcluster)  [unwired: 4 in, 1 out]
        n171 = disable-structure shown="Disabled" {
          disable-tunnel: w387 -> [w402 _]
          frame Disabled {
            n172 = property on="BAT File" class="Path"("StartPath"=w402) -> ()  [unwired: 2 in, 2 out]
            n173 = local write "File List"(i32[] [] ("File List")) -> ()
          }
          frame Enabled {
          }
        }
        n174 = call <vilib>:"Add State(s) to Queue__jki_lib_state_machine.vi"("State(s) in (\"\")"=w400) -> ("States Out"=w399:string)  [unwired: 14 in]
        "Status" <- w392
        "Output" <- w392
      }
      frame "UI: Disable Buttons" {
        # "Do not put any code in this frame.\n(It is a separator no-op. You can make a copy of this frame to create a new UI frame)"
        n175 = control-ref of="Preview"() -> (w411:refnum<vi>)
        n176 = control-ref of="Build"() -> (w410:refnum<vi>)
        n177 = control-ref of="Publish"() -> (w408:refnum<vi>)
        n178 = control-ref of="Clear Notes"() -> (w407:refnum<vi>)
        n179 = control-ref of="Append Notes"() -> (w406:refnum<vi>)
        n180 = control-ref of="Patch +1"() -> (w405:refnum<vi>)
        n181 = control-ref of="Release Notes"() -> (w404:refnum<vi>)
        n182 = control-ref of="BAT"() -> (w403:refnum<vi>)
        n183 = Build Array(w411, w410, w408, w403, w407, w406, w405, w404) -> (w409:refnum<vi>[])
        n184 = for {
          tunnel: w409 -> [w416] mode=indexing
          n185 = property class="Ctl"(reference=w416, "DisabledEnum"=T3."Disabled and Grayed Out" ("Disabled")) -> ()  [unwired: 1 in, 2 out]
        }
        n186 = call <vilib>:"Add State(s) to Queue__jki_lib_state_machine.vi"("State(s) in (\"\")"=w415) -> ("States Out"=w414:string)  [unwired: 14 in]
      }
      frame "UI: Enable Buttons" {
        # "Do not put any code in this frame.\n(It is a separator no-op. You can make a copy of this frame to create a new UI frame)"
        n187 = control-ref of="BAT"() -> (w422:refnum<vi>)
        n188 = Unbundle By Name(w432) -> ("Mode"=w425:T4, "vipb paths"=w423:path[], "vip paths"=w419:path[])
        n189 = control-ref of="Preview"() -> (w434:refnum<vi>)
        n190 = control-ref of="Build"() -> (w433:refnum<vi>)
        n191 = control-ref of="Clear Notes"() -> (w431:refnum<vi>)
        n192 = control-ref of="Append Notes"() -> (w430:refnum<vi>)
        n193 = control-ref of="Patch +1"() -> (w428:refnum<vi>)
        n194 = control-ref of="Release Notes"() -> (w427:refnum<vi>)
        n195 = control-ref of="Publish"() -> (w421:refnum<vi>)
        n196 = Empty Array?(array=w423) -> (empty?=w426:bool)
        n197 = Build Array(w434, w433, w431, w422, w430, w428, w427, w421) -> (w429:refnum<vi>[])
        n198 = Empty Array?(array=w419) -> (empty?=w420:bool)
        n199 = Not(x=w426) -> (.not. x?=w424:bool)
        n200 = Not(x=w420) -> (.not. x?=w418:bool)
        n201 = case shown="\"Build Spec (vipb)\"" w425 {
          tunnel: w429 -> [_ _ w441]
          tunnel: w424 -> [_ _ w440]
          frame "Package (vip)" {
          }
          frame "Project (lvproj)" {
          }
          frame "Build Spec (vipb)" {
            n202 = case shown="True" w440 {
              tunnel: w441 -> [_ w442]
              frame False {
              }
              frame True {
                n203 = for {
                  tunnel: w442 -> [w443] mode=indexing
                  n204 = property class="Ctl"(reference=w443, "DisabledEnum"=T3."Enabled" ("Disabled")) -> ()  [unwired: 1 in, 2 out]
                }
              }
            }
          }
        }
        n205 = case shown="True" w418 {
          frame False {
          }
          frame True {
            n206 = control-ref of="Publish"() -> (w439:refnum<vi>)
            n207 = property class="Bool (strict)"(reference=w439, "DisabledEnum"=T3."Enabled" ("Disabled")) -> ()  [unwired: 1 in, 2 out]
          }
        }
        n208 = call <vilib>:"Add State(s) to Queue__jki_lib_state_machine.vi"("State(s) in (\"\")"=w437) -> ("States Out"=w436:string)  [unwired: 14 in]
      }
      frame "UI: Cursor Set" {
        # "Argument"
        # "Set and Unset Cursor Busy.\n(Usage: \"UI: Cursor Set >> Busy|Idle\")"
        n209 = case shown="\"Busy\"" w445 {
          tunnel: w447 -> [w452 w454]
          tunnel: [w451 w453] -> w446
          frame "Idle", Default {
            n210 = call <vilib>:"Unset Busy.vi"("error in (no error)"=w452) -> ("error out"=w451:errorcluster)  [unwired: 10 in]
          }
          frame "Busy" {
            n211 = call <vilib>:"Set Busy.vi"("error in (no error)"=w454) -> ("error out"=w453:errorcluster)  [unwired: 9 in, 1 out]
          }
        }
        n212 = call <vilib>:"Add State(s) to Queue__jki_lib_state_machine.vi"("State(s) in (\"\")"=w450) -> ("States Out"=w449:string)  [unwired: 14 in]
      }
      frame "UI: Front Panel State" {
        # "Argument"
        # "Set Front Panel Open or Closed\n(Usage: \"UI: Front Panel State >> Open|Close\")"
        n213 = Unbundle By Name(w457) -> ("Core.Current VI Reference"=w456:refnum<vi>)
        n214 = case shown="\"Open\", \"Standard\", Default" w455 {
          tunnel: w459 -> [w467 w482 w493 w506 w519]
          tunnel: [w469 w483 w495 w508 w521] -> w458
          tunnel: w456 -> [w468 w480 w494 w507 w520]
          frame "Open", "Standard", Default {
            w462 = T1."Standard" ("State")
            n215 = property class="VI"(reference=w468, error in=w467) -> (reference out=w465:refnum<vi>, error out=w466:errorcluster, "FP.State"=w464:T1)
            n216 = Not Equal?(x=w464, y=w462) -> (x != y?=w463:bool)
            n217 = case shown="False" w463 {
              tunnel: [w473 w475] -> w469
              tunnel: w466 -> [w472 w475]
              tunnel: w465 -> [w471 _]
              tunnel: w462 -> [w470 _]
              frame True {
                n218 = invoke class="VI" method="FP.Open"(reference=w471, error in=w472, "Activate"=TRUE, "State"=w470) -> (error out=w473:errorcluster)  [unwired: 1 in, 4 out]
              }
              frame False {
              }
            }
          }
          frame "Close", "Closed" {
            n219 = property class="VI"(reference=w480, error in=w482) -> (reference out=w479:refnum<vi>, error out=w481:errorcluster, "FP.State"=w477:T1)
            n220 = Not Equal?(x=w477, y=T1."Closed" ("Front Panel Window:State")) -> (x != y?=w476:bool)
            n221 = case shown="True" w476 {
              tunnel: [w484 w487] -> w483
              tunnel: w481 -> [w484 w486]
              tunnel: w479 -> [_ w485]
              frame False {
              }
              frame True {
                n222 = invoke class="VI" method="FP.Close"(reference=w485, error in=w486) -> (error out=w487:errorcluster)  [unwired: 1 in, 2 out]
              }
            }
          }
          frame "Hidden", "Hide" {
            w488 = T1."Hidden" ("State")
            n223 = property class="VI"(reference=w494, error in=w493) -> (reference out=w491:refnum<vi>, error out=w492:errorcluster, "FP.State"=w490:T1)
            n224 = Not Equal?(x=w490, y=w488) -> (x != y?=w489:bool)
            n225 = case shown="True" w489 {
              tunnel: [w499 w500] -> w495
              tunnel: w492 -> [w498 w500]
              tunnel: w491 -> [w497 _]
              tunnel: w488 -> [w496 _]
              frame True {
                n226 = invoke class="VI" method="FP.Open"(reference=w497, error in=w498, "State"=w496) -> (error out=w499:errorcluster)  [unwired: 2 in, 4 out]
              }
              frame False {
              }
            }
          }
          frame "Minimize", "Minimized" {
            w501 = T1."Minimized" ("State")
            n227 = property class="VI"(reference=w507, error in=w506) -> (reference out=w504:refnum<vi>, error out=w505:errorcluster, "FP.State"=w503:T1)
            n228 = Not Equal?(x=w503, y=w501) -> (x != y?=w502:bool)
            n229 = case shown="True" w502 {
              tunnel: [w512 w513] -> w508
              tunnel: w505 -> [w511 w513]
              tunnel: w504 -> [w510 _]
              tunnel: w501 -> [w509 _]
              frame True {
                n230 = invoke class="VI" method="FP.Open"(reference=w510, error in=w511, "State"=w509) -> (error out=w512:errorcluster)  [unwired: 2 in, 4 out]
              }
              frame False {
              }
            }
          }
          frame "Maximize", "Maximized" {
            w514 = T1."Maximized" ("State")
            n231 = property class="VI"(reference=w520, error in=w519) -> (reference out=w517:refnum<vi>, error out=w518:errorcluster, "FP.State"=w516:T1)
            n232 = Not Equal?(x=w516, y=w514) -> (x != y?=w515:bool)
            n233 = case shown="True" w515 {
              tunnel: [w525 w526] -> w521
              tunnel: w518 -> [w524 w526]
              tunnel: w517 -> [w523 _]
              tunnel: w514 -> [w522 _]
              frame True {
                n234 = invoke class="VI" method="FP.Open"(reference=w523, error in=w524, "State"=w522) -> (error out=w525:errorcluster)  [unwired: 2 in, 4 out]
              }
              frame False {
              }
            }
          }
        }
        n235 = call <vilib>:"Add State(s) to Queue__jki_lib_state_machine.vi"("State(s) in (\"\")"=w461) -> ("States Out"=w460:string)  [unwired: 14 in]
      }
      frame "---------- Macro ----------" {
        # "Do not put any code in this frame.\n(It is a separator no-op. You can make a copy of this frame to create a new Macro frame)"
        n236 = call <vilib>:"Add State(s) to Queue__jki_lib_state_machine.vi"("State(s) in (\"\")"=w530) -> ("States Out"=w529:string)  [unwired: 14 in]
      }
      frame "Macro: Initialize" {
        w531 = "Data: Initialize\nInitialize Core Data\nUI: Initialize\nUI: Front Panel State >> Open\n\nMacro: Read File"  # Data: Initialize Initialize Core Data UI: Initialize UI: Front Panel State >> Open  Macro: Read File
        # "Initialization Macro\n(This is called once, when the VI starts)"
        n237 = call <vilib>:"Add State(s) to Queue__jki_lib_state_machine.vi"("State(s) in Front (\"\")"=w531, "State(s) in (\"\")"=w535) -> ("States Out"=w534:string)  [unwired: 13 in]
      }
      frame "Macro: Read File" {
        # "open"
        # "edit"
        # "Initialization Macro\n(This is called once, when the VI starts)"
        n238 = Equal?(x=w536, y="edit") -> (x = y?=w537:bool)
        n239 = Select(t="UI: Cursor Set >> Busy\nUI: Disable Buttons\n//Data: Choose File List\nData: Read File List\nData: Update Listbox\nUI: Enable Buttons\nUI: Cursor Set >> Idle", s=w537, f="UI: Cursor Set >> Busy\nUI: Disable Buttons\nData: Choose File List\nData: Read File List\nData: Update Listbox\nUI: Enable Buttons\nUI: Cursor Set >> Idle") -> (s? t:f=w541:string)
        n240 = call <vilib>:"Add State(s) to Queue__jki_lib_state_machine.vi"("State(s) in Front (\"\")"=w541, "State(s) in (\"\")"=w545) -> ("States Out"=w544:string)  [unwired: 13 in]
      }
      frame "Macro: Exit" {
        # "Exit Macro\n(This is called once, when the VI exits)"
        n241 = Unbundle By Name(w552) -> ("Core.Close Panel on Exit?"=w551:bool)
        n242 = Select(t="UI: Front Panel State >> Close", s=w551, f="") -> (s? t:f=w548:string)
        n243 = call <vilib>:"Add State(s) to Queue__jki_lib_state_machine.vi"("State(s) in (\"\")"=w548, "State(s) at Back (\"\")"="Data: Cleanup\nExit") -> ("States Out"=w546:string)  [unwired: 13 in]
        n244 = call <vilib>:"Add State(s) to Queue__jki_lib_state_machine.vi"("State(s) in Front (\"\")"=w546, "State(s) in (\"\")"=w555) -> ("States Out"=w554:string)  [unwired: 13 in]
      }
      frame "---------- Action ----------" {
        # "Template Separator\n(You can make a copy of, or modify, this frame)"
        n245 = call <vilib>:"Add State(s) to Queue__jki_lib_state_machine.vi"("State(s) in (\"\")"=w559) -> ("States Out"=w558:string)  [unwired: 14 in]
      }
      frame "Action: Open File" {
        # "Your code here.\n(You can make a copy of, or modify, this frame)"
        n246 = Unbundle By Name(w573) -> ("path to open"=w560:path)
        n247 = Strip Path(path=w560) -> (name=w566:string)  [unwired: 1 out]
        n248 = Format Into String(format string="Opening \"%s\"...", error in=w571, w566) -> (resulting string=w561:string, error out=w563:errorcluster)  [unwired: 1 in]
        n249 = control-ref of="Status"() -> (w564:refnum<vi>)
        n250 = call "Status.vi"("Status Indicator Reference"=w564, "error in (no error)"=w563, "Status"=w561) -> ("error out"=w562:errorcluster)  [unwired: 8 in]
        n251 = Format Into String(format string="cmd /c explorer.exe \"%s\"", error in=w562, w560) -> (resulting string=w569:string, error out=w567:errorcluster)  [unwired: 1 in]
        n252 = call <vilib>:"System Exec.vi"("run minimized? (F)"=TRUE, "error in (no error)"=w567, "command line"=w569) -> ("error out"=w572:errorcluster)  [unwired: 5 in, 3 out]
        n253 = call <vilib>:"Add State(s) to Queue__jki_lib_state_machine.vi"("State(s) in (\"\")"=w575) -> ("States Out"=w574:string)  [unwired: 14 in]
      }
      frame "Action: Open Folder" {
        # "Your code here.\n(You can make a copy of, or modify, this frame)"
        n254 = Unbundle By Name(w579) -> ("selected paths"=w576:path[])
        n255 = for {
          tunnel: w578 -> [w585]
          tunnel: [w583] -> w577
          tunnel: w576 -> [w582] mode=indexing
          n256 = call "Walk Up to Repository.vi"("error in (no error)"=w585, "Build Path"=w582) -> ("error out"=w586:errorcluster, "Repository Path"=w584:path)  [unwired: 8 in]
          n257 = Strip Path(path=w584) -> (name=w592:string)  [unwired: 1 out]
          n258 = Format Into String(format string="Opening \"%s\"...", error in=w586, w592) -> (resulting string=w587:string, error out=w589:errorcluster)  [unwired: 1 in]
          n259 = control-ref of="Status"() -> (w590:refnum<vi>)
          n260 = call "Status.vi"("Status Indicator Reference"=w590, "error in (no error)"=w589, "Status"=w587) -> ("error out"=w588:errorcluster)  [unwired: 8 in]
          n261 = Format Into String(format string="cmd /c explorer.exe \"%s\"", error in=w588, w584) -> (resulting string=w595:string, error out=w593:errorcluster)  [unwired: 1 in]
          n262 = call <vilib>:"System Exec.vi"("run minimized? (F)"=TRUE, "error in (no error)"=w593, "command line"=w595) -> ("error out"=w583:errorcluster)  [unwired: 5 in, 3 out]
        }
        n263 = call <vilib>:"Add State(s) to Queue__jki_lib_state_machine.vi"("State(s) in (\"\")"=w581) -> ("States Out"=w580:string)  [unwired: 14 in]
      }
      frame "Action: Initialize Repository" {
        # "Your code here.\n(You can make a copy of, or modify, this frame)"
        n264 = Unbundle By Name(w607) -> ("config folder"=w604:path, "selected paths"=w605:path[])
        n265 = for {
          tunnel: w606 -> [w620]
          tunnel: w605 -> [w611] mode=indexing
          tunnel: w604 -> [w612]
          tunnel: [w613] -> w603
          tunnel: [w610] -> w602 mode=concatenating
          n266 = Strip Path(path=w611) -> (name=w619:string)  [unwired: 1 out]
          n267 = Format Into String(format string="Initializing \"%s\"...", error in=w620, w619) -> (resulting string=w615:string, error out=w616:errorcluster)  [unwired: 1 in]
          n268 = control-ref of="Status"() -> (w617:refnum<vi>)
          n269 = call "Status.vi"("Status Indicator Reference"=w617, "error in (no error)"=w616, "Status"=w615) -> ("error out"=w614:errorcluster)  [unwired: 8 in]
          n270 = call "Initialize Repository.vi"("config folder"=w612, "error in (no error)"=w614, "Path"=w611) -> ("error out"=w613:errorcluster, "Files Copied"=w610:path[])  [unwired: 7 in]
        }
        n271 = Path To String(path=w602) -> (string=w600:string[])
        n272 = call <vilib>:"1D String Array to Delimited String.vi"("delimiter"="\n", "string array"=w600) -> ("delimited string"=w599:string)  [unwired: 9 in]
        n273 = Format Into String(format string="Files created:\n%s", w599) -> (resulting string=w597:string)  [unwired: 2 in, 1 out]
        n274 = local write "Output"(w597) -> ()
        n275 = call <vilib>:"Add State(s) to Queue__jki_lib_state_machine.vi"("State(s) in (\"\")"=w609) -> ("States Out"=w608:string)  [unwired: 14 in]
      }
      frame "Action: Edit TXT File" {
        # "Your code here.\n(You can make a copy of, or modify, this frame)"
        n276 = Unbundle By Name(w625) -> ("selected paths"=w621:path[])
        n277 = for {
          tunnel: w624 -> [w630]
          tunnel: [w636] -> w623
          tunnel: w622 -> [w632]
          tunnel: w621 -> [w629] mode=indexing
          n278 = call "Walk Up to Repository.vi"("error in (no error)"=w630, "Build Path"=w629) -> ("error out"=w631:errorcluster, "Repository Path"=w635:path)  [unwired: 8 in]
          n279 = Build Path(base path=w635, name or relative path="build support") -> (appended path=w633:path)
          n280 = control-ref of="Status"() -> (w640:refnum<vi>)
          n281 = Build Path(base path=w633, name or relative path=w632) -> (appended path=w628:path)
          n282 = Strip Path(path=w628) -> (name=w642:string)  [unwired: 1 out]
          n283 = Format Into String(format string="Opening \"%s\"...", error in=w631, w642) -> (resulting string=w637:string, error out=w639:errorcluster)  [unwired: 1 in]
          n284 = call "Status.vi"("Status Indicator Reference"=w640, "error in (no error)"=w639, "Status"=w637) -> ("error out"=w638:errorcluster)  [unwired: 8 in]
          n285 = call "Edit Text File.vi"("error in (no error)"=w638, "file path"=w628) -> ("error out"=w636:errorcluster)  [unwired: 9 in]
        }
        n286 = call <vilib>:"Add State(s) to Queue__jki_lib_state_machine.vi"("State(s) in (\"\")"=w627) -> ("States Out"=w626:string)  [unwired: 14 in]
      }
      frame "---------- VIPM ----------" {
        # "Template Separator\n(You can make a copy of, or modify, this frame)"
        n287 = call <vilib>:"Add State(s) to Queue__jki_lib_state_machine.vi"("State(s) in (\"\")"=w646) -> ("States Out"=w645:string)  [unwired: 14 in]
      }
      frame "VIPM: Preview VIPB" {
        # "Your code here.\n(You can make a copy of, or modify, this frame)"
        n288 = Unbundle By Name(w653) -> ("selected paths"=w649:path[])
        n289 = for {
          tunnel: w649 -> [w666] mode=indexing
          tunnel: w652 -> [w661]
          tunnel: [w660] -> w648
          tunnel: [w659] -> w650 mode=indexing
          n290 = Strip Path(path=w666) -> (name=w664:string)  [unwired: 1 out]
          n291 = Format Into String(format string="Reading \"%s\"...", w664) -> (resulting string=w657:string)  [unwired: 2 in, 1 out]
          n292 = control-ref of="Status"() -> (w663:refnum<vi>)
          n293 = call "Status.vi"("Status Indicator Reference"=w663, "error in (no error)"=w661, "Status"=w657) -> ("error out"=w662:errorcluster)  [unwired: 8 in]
          n294 = call <vilib>:"Read VI Package Build Spec_vipm_api.vi"("error in (no error)"=w662, "Path to VIPB File"=w666) -> ("error out"=w658:errorcluster, "VI Package Build Spec Data"=w656:T8)  [unwired: 8 in]
          n295 = call "Format Build Spec Summary.vi"("error in (no error)"=w658, "VI Package Build Spec Data"=w656) -> ("error out"=w660:errorcluster, "VIPB Preview"=w659:string)  [unwired: 8 in]
        }
        n296 = call <vilib>:"1D String Array to Delimited String.vi"("delimiter"="\r\n", "string array"=w650) -> ("delimited string"=w647:string)  [unwired: 9 in]
        n297 = local write "Output"(w647) -> ()
        n298 = call <vilib>:"Add State(s) to Queue__jki_lib_state_machine.vi"("State(s) in (\"\")"=w655) -> ("States Out"=w654:string)  [unwired: 14 in]
      }
      frame "VIPM: Increment Patch" {
        # "Your code here.\n(You can make a copy of, or modify, this frame)"
        n299 = Unbundle By Name(w670) -> ("selected paths"=w667:path[])
        n300 = for {
          tunnel: w667 -> [w678] mode=indexing
          tunnel: w669 -> [w676]
          tunnel: [w673] -> w668
          n301 = Strip Path(path=w678) -> (name=w679:string)  [unwired: 1 out]
          n302 = Format Into String(format string="Updating \"%s\"...", w679) -> (resulting string=w674:string)  [unwired: 2 in, 1 out]
          n303 = control-ref of="Status"() -> (w677:refnum<vi>)
          n304 = call "Status.vi"("Status Indicator Reference"=w677, "error in (no error)"=w676, "Status"=w674) -> ("error out"=w675:errorcluster)  [unwired: 8 in]
          n305 = call "Increment Version Patch.vi"("error in (no error)"=w675, "path"=w678) -> ("error out"=w673:errorcluster)  [unwired: 9 in]
        }
        n306 = call <vilib>:"Add State(s) to Queue__jki_lib_state_machine.vi"("State(s) in (\"\")"=w672) -> ("States Out"=w671:string)  [unwired: 14 in]
      }
      frame "VIPM: Increment Minor" {
        # "Your code here.\n(You can make a copy of, or modify, this frame)"
        n307 = Unbundle By Name(w684) -> ("selected paths"=w681:path[])
        n308 = for {
          tunnel: w681 -> [w692] mode=indexing
          tunnel: w683 -> [w690]
          tunnel: [w687] -> w682
          n309 = Strip Path(path=w692) -> (name=w693:string)  [unwired: 1 out]
          n310 = Format Into String(format string="Updating \"%s\"...", w693) -> (resulting string=w688:string)  [unwired: 2 in, 1 out]
          n311 = control-ref of="Status"() -> (w691:refnum<vi>)
          n312 = call "Status.vi"("Status Indicator Reference"=w691, "error in (no error)"=w690, "Status"=w688) -> ("error out"=w689:errorcluster)  [unwired: 8 in]
          n313 = call "Increment Version Minor.vi"("error in (no error)"=w689, "selected path"=w692) -> ("error out"=w687:errorcluster)  [unwired: 9 in]
        }
        n314 = call <vilib>:"Add State(s) to Queue__jki_lib_state_machine.vi"("State(s) in (\"\")"=w686) -> ("States Out"=w685:string)  [unwired: 14 in]
      }
      frame "VIPM: Clear Notes" {
        # "Your code here.\n(You can make a copy of, or modify, this frame)"
        n315 = Unbundle By Name(w701) -> ("selected paths"=w696:path[])
        n316 = for {
          tunnel: w696 -> [w712] mode=indexing
          tunnel: w700 -> [w710]
          tunnel: [w708] -> w695
          tunnel: [w707] -> w698 mode=indexing
          n317 = Strip Path(path=w712) -> (name=w713:string)  [unwired: 1 out]
          n318 = Format Into String(format string="Updating \"%s\"...", w713) -> (resulting string=w704:string)  [unwired: 2 in, 1 out]
          n319 = control-ref of="Status"() -> (w711:refnum<vi>)
          n320 = call "Status.vi"("Status Indicator Reference"=w711, "error in (no error)"=w710, "Status"=w704) -> ("error out"=w709:errorcluster)  [unwired: 8 in]
          n321 = call "Clear Change Log.vi"("error in (no error)"=w709, "selected path"=w712) -> ("error out"=w706:errorcluster, "VI Package Build Spec Data"=w705:T8)  [unwired: 8 in]
          n322 = call "Format Build Spec Summary.vi"("error in (no error)"=w706, "VI Package Build Spec Data"=w705) -> ("error out"=w708:errorcluster, "VIPB Preview"=w707:string)  [unwired: 8 in]
        }
        n323 = call <vilib>:"1D String Array to Delimited String.vi"("delimiter"="\r\n", "string array"=w698) -> ("delimited string"=w697:string)  [unwired: 9 in]
        n324 = local write "Output"(w697) -> ()
        n325 = call <vilib>:"Add State(s) to Queue__jki_lib_state_machine.vi"("State(s) in (\"\")"=w703) -> ("States Out"=w702:string)  [unwired: 14 in]
      }
      frame "VIPM: Append Notes" {
        # "Your code here.\n(You can make a copy of, or modify, this frame)"
        n326 = Unbundle By Name(w722) -> ("selected paths"=w716:path[])
        n327 = for {
          tunnel: w716 -> [w734] mode=indexing
          tunnel: w721 -> [w731]
          tunnel: [w729] -> w715
          tunnel: [w728] -> w718 mode=indexing
          tunnel: "Release Notes" -> [w727]
          n328 = Strip Path(path=w734) -> (name=w735:string)  [unwired: 1 out]
          n329 = Format Into String(format string="Updating \"%s\"...", w735) -> (resulting string=w726:string)  [unwired: 2 in, 1 out]
          n330 = control-ref of="Status"() -> (w733:refnum<vi>)
          n331 = call "Status.vi"("Status Indicator Reference"=w733, "error in (no error)"=w731, "Status"=w726) -> ("error out"=w732:errorcluster)  [unwired: 8 in]
          n332 = call "Append to Change Log.vi"("error in (no error)"=w732, "Release Notes"=w727, "path"=w734) -> ("error out"=w730:errorcluster, "VI Package Build Spec Data"=w725:T8)  [unwired: 7 in]
          n333 = call "Format Build Spec Summary.vi"("error in (no error)"=w730, "VI Package Build Spec Data"=w725) -> ("error out"=w729:errorcluster, "VIPB Preview"=w728:string)  [unwired: 8 in]
        }
        n334 = call <vilib>:"1D String Array to Delimited String.vi"("delimiter"="\r\n", "string array"=w718) -> ("delimited string"=w717:string)  [unwired: 9 in]
        n335 = local write "Output"(w717) -> ()
        n336 = call <vilib>:"Add State(s) to Queue__jki_lib_state_machine.vi"("State(s) in (\"\")"=w724) -> ("States Out"=w723:string)  [unwired: 14 in]
      }
      frame "VIPM: Build" {
        # "Template Separator\n(You can make a copy of, or modify, this frame)"
        n337 = Unbundle By Name(w743) -> ("selected paths"=w739:path[])
        n338 = control-ref of="Status"() -> (w741:refnum<vi>)
        n339 = for {
          tunnel: w739 -> [w761] mode=indexing
          tunnel: [w768] -> w740 mode=indexing if=w762
          tunnel: w738 -> [w766]
          tunnel: [w747] -> w737
          tunnel: w741 -> [w757]
          n340 = Strip Path(path=w761) -> (name=w755:string)  [unwired: 1 out]
          n341 = Format Into String(format string="\nPatrick Builder Start: %s", w755) -> (resulting string=w753:string)  [unwired: 2 in, 1 out]
          n342 = call "Status.vi"("Status Indicator Reference"=w757, "error in (no error)"=w766, "Status"=w753) -> ("error out"=w760:errorcluster)  [unwired: 8 in]
          n343 = call "Status.vi"("Status Indicator Reference"=w757, "error in (no error)"=w760, "Status"="Git Flow Release Start" ("format string")) -> ("error out"=w759:errorcluster)  [unwired: 8 in]
          n344 = local read "tag prefix"() -> (w754:string)
          n345 = call "Macro Start Release.vi"("tag prefix (level1/level2)"=w754, "error in (no error)"=w759, "VIPB Path"=w761) -> ("error out"=w749:errorcluster, "Git out"=w767:refnum<class "Git.lvclass">)  [unwired: 7 in]
          n346 = call "Status.vi"("Status Indicator Reference"=w757, "error in (no error)"=w749, "Status"="VIPM Building..." ("format string")) -> ("error out"=w765:errorcluster)  [unwired: 8 in]
          n347 = call <vilib>:"Build VI Package_vipm_api.vi"("error in (no error)"=w765, "Path to VIPB File"=w761) -> ("error out"=w763:errorcluster, "Build Output"=w768:path)  [unwired: 8 in]
          n348 = call "Status.vi"("Status Indicator Reference"=w757, "error in (no error)"=w763, "Status"="Git Flow Release Finish" ("format string")) -> ("error out"=w764:errorcluster)  [unwired: 8 in]
          n349 = call "Macro Finish Release.vi"("error in (no error)"=w764, "Git in"=w767) -> ("error out"=w758:errorcluster, "standard output"=w748:string)  [unwired: 7 in, 1 out]
          n350 = call "Status.vi"("Status Indicator Reference"=w757, "error in (no error)"=w758, "Status"=w748) -> ("error out"=w747:errorcluster)  [unwired: 8 in]
          n351 = Not(x=w747) -> (.not. x?=w762:bool)
        }
        n352 = Bundle By Name(cluster=w743, "vip paths"=w740) -> (w744:T5)
        n353 = call <vilib>:"Add State(s) to Queue__jki_lib_state_machine.vi"("State(s) in Front (\"\")"="" ("State(s) at Back (\"\")"), "State(s) in (\"\")"=w746) -> ("States Out"=w745:string)  [unwired: 13 in]
      }
      frame "VIPM: Create Build File" {
        # "Template Separator\n(You can make a copy of, or modify, this frame)"
        n354 = Unbundle By Name(w769) -> ("selected paths"=w774:path[])
        n355 = control-ref of="Status"() -> (w775:refnum<vi>)
        n356 = for {
          tunnel: w774 -> [w783] mode=indexing
          tunnel: w773 -> [w787]
          tunnel: [w780] -> w772
          tunnel: w775 -> [w786]
          tunnel: [w781] -> w771 mode=indexing
          n357 = Strip Path(path=w783) -> (stripped path=w782:path, name=w779:string)
          n358 = Format Into String(format string="Find %s repository root", w779) -> (resulting string=w784:string)  [unwired: 2 in, 1 out]
          n359 = call "Status.vi"("Status Indicator Reference"=w786, "error in (no error)"=w787, "Status"=w784) -> ("error out"=w780:errorcluster)  [unwired: 8 in]
          n360 = Strip Path(path=w782) -> (stripped path=w781:path)  [unwired: 1 out]
        }
        n361 = Bundle By Name(cluster=w769, "repository paths"=w771) -> (w770:T5)
        n362 = call <vilib>:"Add State(s) to Queue__jki_lib_state_machine.vi"("State(s) in Front (\"\")"="" ("State(s) at Back (\"\")"), "State(s) in (\"\")"=w778) -> ("States Out"=w777:string)  [unwired: 13 in]
      }
      frame "VIPM: Create Build All File" {
        # "Template Separator\n(You can make a copy of, or modify, this frame)"
        n363 = control-ref of="Status"() -> (w798:refnum<vi>)
        n364 = Unbundle By Name(w790) -> ("config folder"=w792:path, "repository paths"=w797:path[])
        n365 = call "Status.vi"("Status Indicator Reference"=w798, "error in (no error)"=w795, "Status"="Creating build_all.bat") -> ("error out"=w794:errorcluster)  [unwired: 8 in]
        n366 = call "Create build_all.bat.vi"("template folder"=w792, "error in (no error)"=w794, "repository paths"=w797) -> ("error out"=w788:errorcluster, "resulting string"=w796:string, "build_all.bat path"=w789:path)  [unwired: 6 in]
        n367 = local write "BAT File"(w789) -> ()
        n368 = local write "Output"(w796) -> ()
        n369 = Bundle By Name(cluster=w790, ".bat path"=w789) -> (w791:T5)
        n370 = call <vilib>:"Add State(s) to Queue__jki_lib_state_machine.vi"("State(s) in (\"\")"=w800) -> ("States Out"=w799:string)  [unwired: 14 in]
      }
      frame "VIPM: Run BAT File" {
        # "Template Separator\n(You can make a copy of, or modify, this frame)"
        n371 = Unbundle By Name(w812) -> (".bat path"=w802:path)
        n372 = Strip Path(path=w802) -> (name=w803:string)  [unwired: 1 out]
        n373 = control-ref of="Status"() -> (w804:refnum<vi>)
        n374 = Format Into String(format string="\nrunning %s" ("Status"), w803) -> (resulting string=w808:string)  [unwired: 2 in, 1 out]
        n375 = control-ref of="Status"() -> (w815:refnum<vi>)
        n376 = Format Into String(format string="\"%s\"", w802) -> (resulting string=w806:string)  [unwired: 2 in, 1 out]
        n377 = call "Status.vi"("Status Indicator Reference"=w804, "error in (no error)"=w820, "Status"=w808) -> ("error out"=w811:errorcluster)  [unwired: 8 in]
        n378 = call ".NET Terminal.vi"("command line"="cmd.exe", "Status"=w815, "error in (no error)"=w811, "StdIn"=w806) -> ("error out"=w801:errorcluster, "StdOut"=w805:string)  [unwired: 5 in, 1 out]
        n379 = call <vilib>:"Delimited String to 1D String Array.vi"("delimiter"="\n", "delimited string"=w805) -> ("string array"=w817:string[])  [unwired: 9 in]
        n380 = for {
          tunnel: w817 -> [w827] mode=indexing
          tunnel: "BUILD_OUTPUT=\\\"(.*)\\\"" ("regular expression") -> [w826]
          tunnel: [w825] -> w814 mode=indexing if=w823
          n381 = xnode "Match Regular Expression"("input string"=w827, "regular expression"=w826) -> ("offset past match"=w824:i32, "submatch 1"=w825:string)  [unwired: 4 in, 4 out]
          n382 = Greater Or Equal To 0?(x=w824) -> (x >= 0?=w823:bool)
        }
        n383 = String To Path(string=w814) -> (path=w810:path[])
        n384 = Bundle By Name(cluster=w812, "vip paths"=w810) -> (w813:T5)
        n385 = call <vilib>:"Add State(s) to Queue__jki_lib_state_machine.vi"("State(s) in (\"\")"=w822) -> ("States Out"=w821:string)  [unwired: 14 in]
      }
      frame "VIPM: Publish" {
        # "ths is being phased out?"
        # "Template Separator\n(You can make a copy of, or modify, this frame)"
        n386 = control-ref of="Status"() -> (w949:refnum<vi>)
        n387 = Unbundle By Name(w952) -> ("vip paths"=w951:path[])
        n388 = call "Publish Packages to Package Repository.vi"("String in"=w949, "error in (no error)"=w948, "vip paths"=w951) -> ("error out"=w947:errorcluster, "Repository Folder Location"=w946:path, "Package Names Published"=w944:string[])  [unwired: 6 in]
        n389 = Empty Array?(array=w944) -> (empty?=w945:bool)
        n390 = case shown="False" w945 {
          tunnel: [w971 w972] -> w950
          tunnel: w949 -> [w958 _]
          tunnel: w947 -> [w957 w972]
          tunnel: w946 -> [w956 _]
          tunnel: w944 -> [w955 _]
          frame False {
            n391 = call <vilib>:"1D String Array to Delimited String.vi"("delimiter"="\n", "string array"=w955) -> ("delimited string"=w959:string)  [unwired: 9 in]
            n392 = call "Macro Init.vi"("error in (no error)"=w957, "Repository Path"=w956) -> ("error out"=w965:errorcluster, "Git out"=w964:refnum<class "Git.lvclass">)  [unwired: 8 in]
            n393 = call "Macro Add.vi"("error in (no error)"=w965, "Git in"=w964) -> ("error out"=w962:errorcluster, "Git out"=w963:refnum<class "Git.lvclass">)  [unwired: 8 in]
            n394 = Format Into String(format string="Patrick Builder publish packages:\n%s", w959) -> (resulting string=w966:string)  [unwired: 2 in, 1 out]
            n395 = call "Macro Commit.vi"("error in (no error)"=w962, "msg"=w966, "Git in"=w963) -> ("error out"=w967:errorcluster, "Git out"=w969:refnum<class "Git.lvclass">)  [unwired: 7 in]
            n396 = call "Macro Push and Push Tags.vi"("error in (no error)"=w967, "Git in"=w969) -> ("error out"=w968:errorcluster, "std out"=w961:string)  [unwired: 7 in, 1 out]
            n397 = call "Status.vi"("Status Indicator Reference"=w958, "error in (no error)"=w968, "Status"=w961) -> ("error out"=w971:errorcluster)  [unwired: 8 in]
          }
          frame True {
          }
        }
        n398 = call <vilib>:"Add State(s) to Queue__jki_lib_state_machine.vi"("State(s) in (\"\")"=w954) -> ("States Out"=w953:string)  [unwired: 14 in]
      }
      frame "---------- git ----------" {
        # "Template Separator\n(You can make a copy of, or modify, this frame)"
        n399 = call <vilib>:"Add State(s) to Queue__jki_lib_state_machine.vi"("State(s) in (\"\")"=w976) -> ("States Out"=w975:string)  [unwired: 14 in]
      }
      frame "---------- Sequence ----------" {
        # "Template Separator\n(You can make a copy of, or modify, this frame)"
        n400 = call <vilib>:"Add State(s) to Queue__jki_lib_state_machine.vi"("State(s) in (\"\")"=w980) -> ("States Out"=w979:string)  [unwired: 14 in]
      }
    }
  }
  n401 = control-ref of="Status"() -> ()  [unwired: 1 out]
  n402 = disable-structure shown="Disabled" {
    frame Disabled {
      n403 = call <vilib>:"Read VI Package Build Spec_vipm_api.vi"() -> ()  [unwired: 10 in, 2 out]
    }
    frame Enabled {
    }
  }
